vi "DAC Run.vi"(8 "error in":errorcluster, 11 "DAC HeatFlow Load dU in":refnum<class "DAC HeatFlow Load dU.lvclass">) -> (0 "error out":errorcluster, 3 "DAC HeatFlow Load dU out":refnum<class "DAC HeatFlow Load dU.lvclass">)   [LabVIEW 2019, in "DAC.lvlib" / "DAC HeatFlow Load dU.lvclass"]
uses:
  DAC HeatFlow Load dU.lvclass
  C:/Users/krio/Documents/LV_Projects/test-stand/App/DAC/DAC.lvclass
  DAC.lvclass/DAC.ctl
  DAC HeatFlow Load dU.lvclass/DAC HeatFlow Load dU.ctl
  <vilib>/DAQmx/read.llb/DAQmx Read (Analog DBL 1Chan 1Samp).vi
  <vilib>/DAQmx/miscellaneous.llb/DAQmx Fill In Error Info.vi
  DAC.lvclass
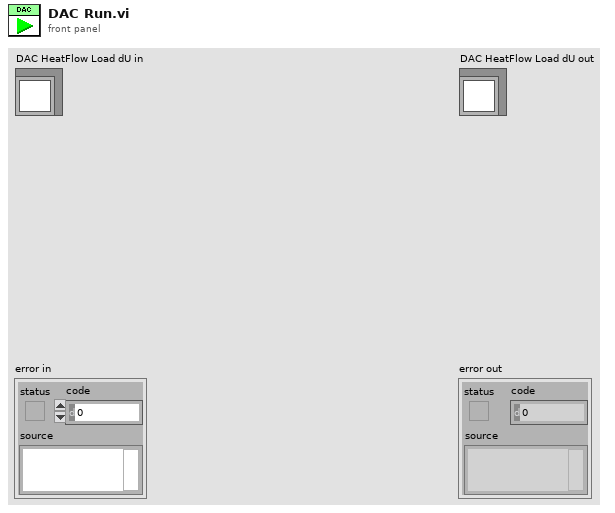
[diagram p1: front panel]
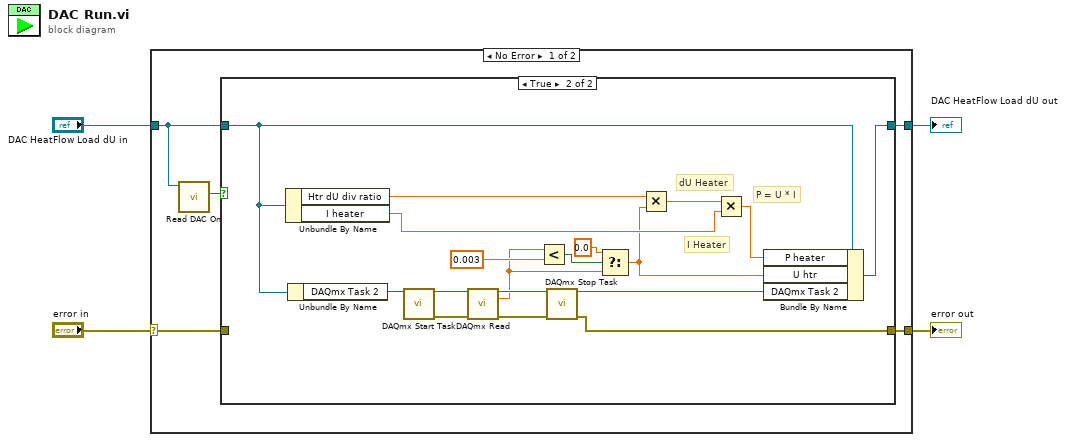
[diagram p0: block diagram]
diagram:
  n1 = case shown="No Error" "error in" {
    selector: "error in" -> [w7 w31]
    tunnel: [w6 w31] -> w2
    tunnel: [w8 w30] -> w1
    tunnel: "DAC HeatFlow Load dU in" -> [w5 w30]
    frame No Error {
      n2 = call "Read DAC On.vi"("DAC in"=w5) -> ("DAC On"=w9:bool)  [unwired: 8 in, 2 out]
      n3 = case shown="True" w9 {
        tunnel: w5 -> [w11 w17]
        tunnel: [w11 w24] -> w8
        tunnel: w7 -> [w10 _]
        tunnel: [w10 w22] -> w6
        frame False {
        }
        frame True {
          # "I Heater"
          # "dU Heater"
          # "P = U * I"
          n4 = Unbundle By Name(w17) -> ("Htr dU div ratio"=w19:dbl, "I heater"=w18:dbl)
          n5 = Unbundle By Name(w17) -> ("DAQmx Task 2"=w29:refnum<k21>)
          n6 = call <vilib>:"DAQmx Start Task.vi"("task/channels in"=w29) -> ("task out"=w28:refnum<k21>, "error out"=w26:errorcluster)  [unwired: 13 in]
          n7 = call-poly <vilib>:"DAQmx Read.vi"("task/channels in"=w28, "error in"=w26) -> ("task out"=w27:refnum<k21>, "data"=w12:dbl, "error out"=w25:errorcluster)  [unwired: 11 in]
          n8 = Less?(x=w12, y=0.003) -> (x < y?=w15:bool)
          n9 = call <vilib>:"DAQmx Stop Task.vi"("task/channels in"=w27, "error in"=w25) -> ("task out"=w23:refnum<k21>, "error out"=w22:errorcluster)  [unwired: 12 in]
          n10 = Select(t=0.0, s=w15, f=w12) -> (s? t:f=w13:dbl)
          n11 = Multiply(x=w19, y=w13) -> (x*y=w21:dbl)
          n12 = Multiply(x=w21, y=w18) -> (x*y=w20:dbl)
          n13 = Bundle By Name(cluster=w17, "P heater"=w20, "U htr"=w13, "DAQmx Task 2"=w23) -> (w24:refnum<class "DAC HeatFlow Load dU.lvclass">)
        }
      }
    }
    frame Error {
    }
  }
  "error out" <- w2
  "DAC HeatFlow Load dU out" <- w1
